vi "SetDigitalOutputState.vi"(8 "error in":errorcluster, 9 "Pin State":bool, 10 "Pin Index":u8, 11 "comport in":refnum<visa-resource-name>) -> (0 "error out":errorcluster={"status"=TRUE, "code"=-1073807339, "source"="VISA Read in FirmataClient.lvlib:Initialize.vi"}, 3 "comport out":refnum<visa-resource-name>)   [LabVIEW 2020, in "FirmataClient.lvlib"]
doc: "Builds and Sends a message according to the Firmata Protocol Requirements. \n- https://github.com/firmata/protocol\n- https://github.com/firmata/protocol/blob/master/protocol.md"
uses:
  FirmataClient.lvlib
  controls/FirmataPinModes.ctl
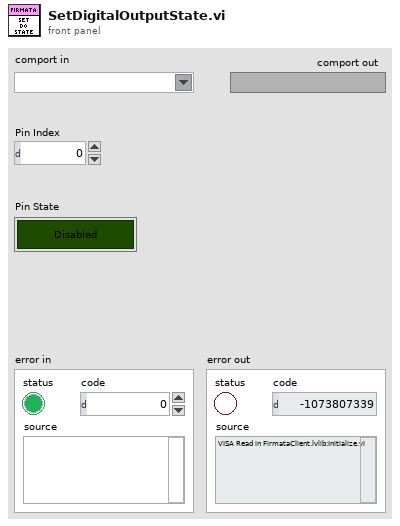
[diagram p1: front panel]
types:
  T1 = typedef "FirmataClient.lvlib/FirmataPinModes.ctl" = enum16{"DigitalInput", "DigitalOutput", "AnalogInput", "PWM", "Servo", "Shift", "I2C", "OneWire", "Stepper", "Encoder", "Serial", "InputPullup", "Extended.SPI", "Extended.Sonar", "Extended.Tone", "Extended.DHT"}
  T2 = typedef "FirmataClient.lvlib/FirmataProtocolConstants.ctl" = u16
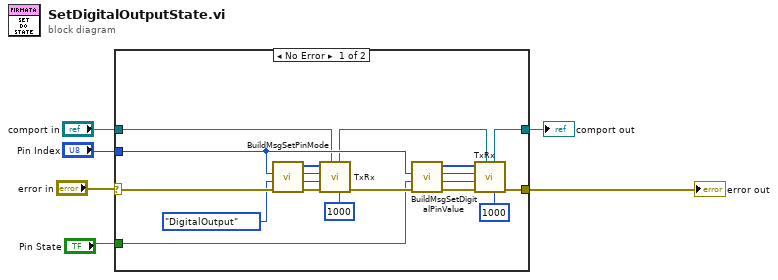
[diagram p0: block diagram]
diagram:
  n1 = case shown="No Error" "error in" {
    selector: "error in" -> [w19 w27]
    tunnel: [w20 w27] -> w5
    tunnel: "Pin Index" -> [w17 _]
    tunnel: "Pin State" -> [w18 _]
    tunnel: [w7 w26] -> w2
    tunnel: "comport in" -> [w9 w26]
    frame No Error {
      n2 = call "BuildMsgSetPinMode.vi"("error in"=w19, "Pin Mode"=FirmataPinModes."DigitalOutput", "Pin Index"=w17) -> ("error out"=w23:errorcluster, "ReplyLength"=w14:i32, "ReplyFirstByte"=w15:T2, "SetPinModeMessage"=w16:u8[])  [unwired: 5 in]
      n3 = call "TxRx.vi"("Timeout"=u32 1000, "comport in"=w9, "error in"=w23, "Expected Reply Length"=w14, "ReplyFirstByte"=w15, "MessageToSend"=w16) -> ("error out"=w21:errorcluster, "comport out"=w8:refnum<visa-resource-name>)  [unwired: 1 in, 3 out]
      n4 = call "BuildMsgSetDigitalPinValue.vi"("error in"=w21, "Pin Value"=w18, "Pin Index"=w17) -> ("error out"=w25:errorcluster, "ReplyLength"=w12:i32, "ReplyFirstByte"=w11:T2, "DigitalPinValueMessage"=w10:u8[])  [unwired: 5 in]
      n5 = call "TxRx.vi"("Timeout"=u32 1000, "comport in"=w8, "error in"=w25, "Expected Reply Length"=w12, "ReplyFirstByte"=w11, "MessageToSend"=w10) -> ("error out"=w20:errorcluster, "comport out"=w7:refnum<visa-resource-name>)  [unwired: 1 in, 3 out]
    }
    frame Error {
    }
  }
  "error out" <- w5
  "comport out" <- w2
